vi "SD Wait for Ready.vi"(0 "Notifier Name":string, 11 "Error In":errorcluster) -> (4 "Notifier Name Out":string, 8 "Ready?":bool, 15 "Error Out":errorcluster)   [LabVIEW 2020]
uses:
  Device Library/Spinning Disk/Spinning Disk Type Defs/SD Notifer Data.ctl
  Device Library/Spinning Disk/Spinning Disk Type Defs/SD Actions.ctl
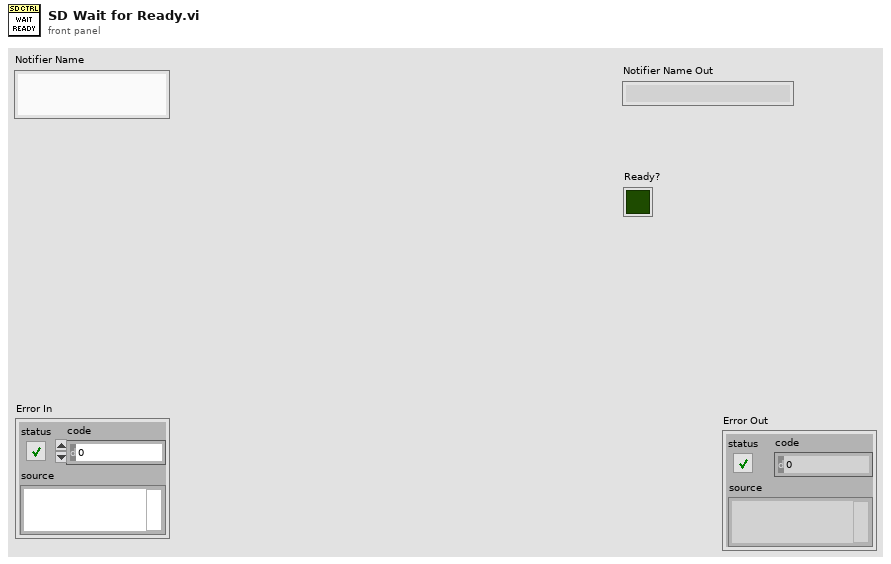
[diagram p1: front panel]
types:
  T1 = typedef "SD Notifer Data.ctl" = cluster{"Actions":T2, "Disk On?":bool, "Dichroic Pos.":i32, "Filter Wheel Pos.":i32, "Disk Pos.":i32, "Recived":bool, "Num Pos":i32[]}
  T2 = typedef "SD Actions.ctl" = enum16{"Status", "Get All Pos.", "Get Num. Pos.", "Home All", "Set Filter Wheel Pos.", "Set Disk Pos.", "Set Dichroic Pos.", "Disk On", "Disk Off", "Quit"}
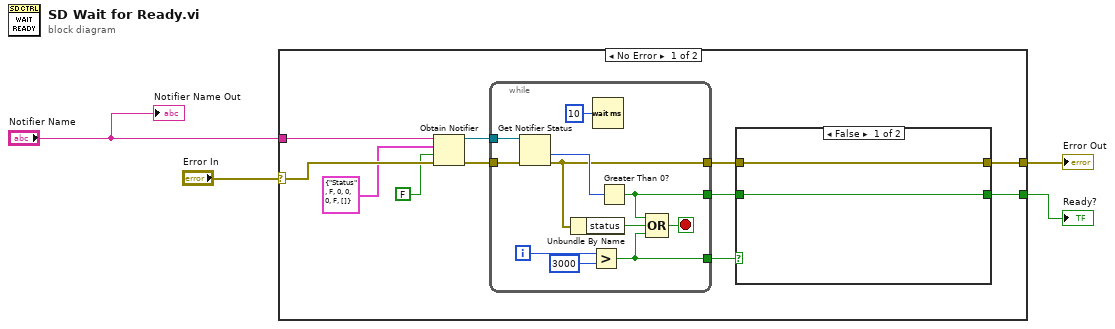
[diagram p0: block diagram]
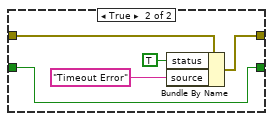
[diagram p2: hidden frame]
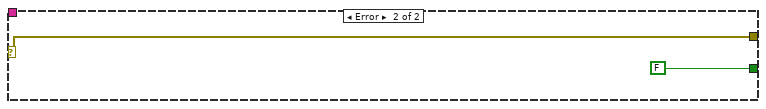
[diagram p3: hidden frame]
diagram:
  n1 = case shown="No Error" "Error In" {
    selector: "Error In" -> [w14 w35]
    tunnel: "Notifier Name" -> [w15 _]
    tunnel: [w13 FALSE] -> w3
    tunnel: [w12 w35] -> w2
    frame No Error {
      n2 = Obtain Notifier(name (unnamed)=w15, notification data type=T1 {"Actions"=enum."Status", "Disk On?"=FALSE, "Dichroic Pos."=0, "Filter Wheel Pos."=0, "Disk Pos."=0, "Recived"=FALSE, "Num Pos"=[]} ("SD Notifier Data"), create if not found? (T)=FALSE, error in (no error)=w14) -> (notifier out=w9:refnum<notifier>, error out=w8:errorcluster)  [unwired: 1 out]
      n3 = while {
        tunnel: w9 -> [w33]
        tunnel: w8 -> [w32]
        tunnel: [w30] -> w5
        tunnel: [w24] -> w6
        tunnel: [w23] -> w7
        i -> [w28]
        stop <- w25 stop-if-true
        n4 = Get Notifier Status(notifier=w33, error in (no error)=w32) -> (# waiting=w31:i32, error out=w30:errorcluster)  [unwired: 3 out]
        n5 = Unbundle By Name(w30) -> ("status"=w26:bool)
        n6 = Greater?(x=w28, y=3000) -> (0:w23:bool)
        n7 = Wait (ms)(milliseconds to wait=u32 10) -> ()  [unwired: 1 out]
        n8 = Greater Than 0?(x=w31) -> (x > 0?=w24:bool)
        n9 = Compound Arithmetic op=OR(w24, w26, w23) -> (w25:bool)
      }
      n10 = case shown="False" w7 {
        tunnel: w6 -> [w17 w18]
        tunnel: [w17 w18] -> w13
        tunnel: w5 -> [w16 w22]
        tunnel: [w16 w20] -> w12
        frame False {
        }
        frame True {
          n11 = Bundle By Name(cluster=w22, "status"=TRUE, "source"="Timeout Error") -> (w20:errorcluster)
        }
      }
    }
    frame Error {
    }
  }
  "Error Out" <- w2
  "Ready?" <- w3
  "Notifier Name Out" <- "Notifier Name"
